vi "Found shot match.vi"(8 "error in (no error)":errorcluster, 9 "Shot data":T1, 10 "Idot match record":T2, 11 "Cap Bank Server in":refnum<class "Cap Bank Server.lvclass">) -> (0 "error out":errorcluster, 3 "Cap Bank Server out":refnum<class "Cap Bank Server.lvclass">)   [LabVIEW 2015, in "Cap Bank Server.lvclass"]
uses:
  Cap Bank Server.lvclass
  Idot match record.ctl
  User Cap Bank/Labview/Library/Shot data.ctl
  File/Controls/File formats.ctl
  <vilib>/ActorFramework/Actor/Actor.lvclass/Actor.ctl
  <vilib>/ActorFramework/Message Enqueuer/Message Enqueuer.lvclass/Message Enqueuer.ctl
  Cap Bank Server.lvclass/Cap Bank Server.ctl
  Mag Lab Measure Controller Messages/Log Status Update Msg/Log Status Update Msg.lvclass/Log Status Update Msg.ctl
  <vilib>/ActorFramework/Message Enqueuer/Init from Existing Queue.vi
  <vilib>/ActorFramework/Message Enqueuer/Enqueue.vi
  <vilib>/ActorFramework/Message Priority Queue/Priority Enqueue.vi
  <vilib>/ActorFramework/Message Enqueuer/Message Enqueuer.lvclass
  Mag Lab Measure Controller Messages/Log Status Update Msg/Log Status Update Msg.lvclass
  <vilib>/ActorFramework/Actor/Actor.lvclass
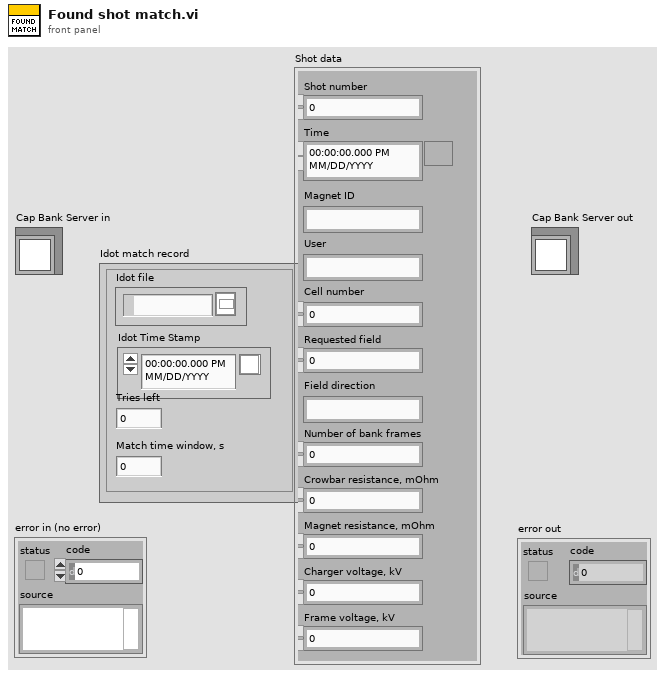
[diagram p1: front panel]
types:
  T1 = typedef "Shot data.ctl" = cluster{"Shot number":i32, "Time":timestamp, "Magnet ID":string, "User":string, "Cell number":i32, "Requested field":dbl, "Field direction":string, "Number of bank frames":i32, "Crowbar resistance, mOhm":dbl, "Magnet resistance, mOhm":dbl, "Charger voltage, kV":dbl, "Frame voltage, kV":dbl}
  T2 = typedef "Idot match record.ctl" = cluster{"Idot file":path, "Idot Time Stamp":timestamp, "Tries left":i32, "Match time window, s":dbl}
  T3 = typedef "File formats.ctl" = enum16{"TDMS", "ASCII", "BINARY"}
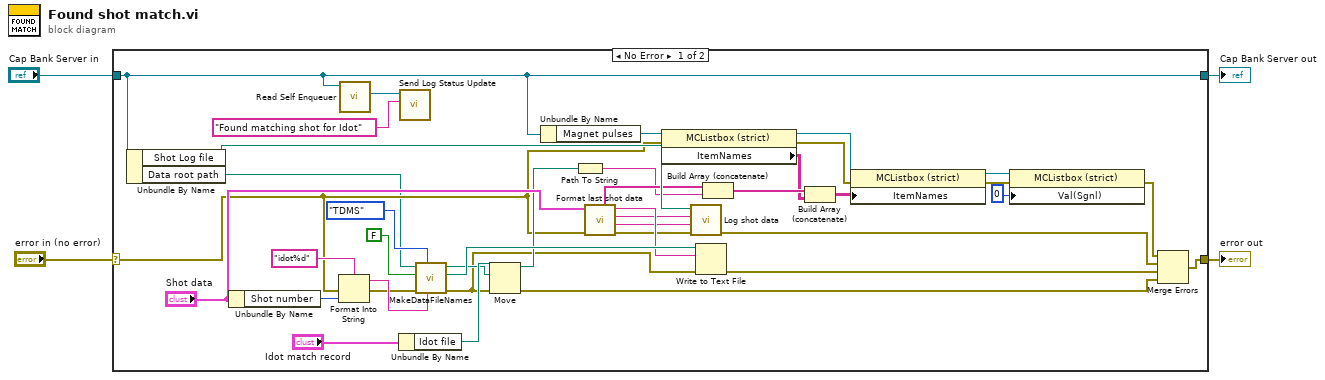
[diagram p0: block diagram]
diagram:
  n1 = case shown="No Error" "error in (no error)" {
    selector: "error in (no error)" -> [w13 w45]
    tunnel: [w26 w45] -> w3
    tunnel: [w23 w44] -> w1
    tunnel: "Cap Bank Server in" -> [w23 w44]
    frame No Error {
      n2 = Unbundle By Name(w23) -> ("Shot Log file"=w29:path, "Data root path"=w5:path)
      n3 = Unbundle By Name("Shot data") -> ("Shot number"=w34:i32)
      n4 = Format Into String(format string="idot%d", error in=w13, w34) -> (resulting string=w41:string, error out=w35:errorcluster)  [unwired: 1 in]
      n5 = call <vilib>:"Read Self Enqueuer.vi"("Actor"=w23) -> ("Self Enqueuer"=w25:refnum<class "Message Enqueuer.lvclass">)  [unwired: 10 in]
      n6 = Unbundle By Name("Idot match record") -> ("Idot file"=w32:path)
      n7 = call "Send Log Status Update.vi"("Status"="Found matching shot for Idot", "Message Enqueuer"=w25) -> ()  [unwired: 8 in, 2 out]
      n8 = call "MakeDataFileNames.vi"("File Prefix"=w41, "File format"=File_formats."TDMS", "Error In"=w35, "Generate Index"=FALSE, "Root Data Folder"=w5) -> ("Error Out"=w16:errorcluster, "Settings File Path"=w39:path, "Data File  Path"=w31:path)  [unwired: 3 in, 1 out]
      n9 = Move(source path=w32, error in=w16, 10:w31) -> (error out=w27:errorcluster, 3:w21:path)  [unwired: 2 in, 1 out]
      n10 = Unbundle By Name(w23) -> ("Magnet pulses"=w22:refnum<vi>)
      n11 = Path To String(path=w21) -> (string=w19:string)
      n12 = call "Format last shot data.vi"("error in (no error)"=w13, "Shot data"="Shot data") -> ("error out"=w15:errorcluster, "Spreadsheet header string"=w36:string, "Spreadsheet shot string"=w37:string, "Formated shot data"=w38:string, "Listbox entry"=w20:string[])  [unwired: 5 in]
      n13 = property class="MCListbox (strict)"(reference=w22, error in=w13) -> (reference out=w18:refnum<vi>, error out=w17:errorcluster, "ItemNames"=w11:string[][])
      n14 = call "Log shot data.vi"("error in (no error)"=w15, "Spreadsheet header string"=w36, "Spreadsheet shot string"=w37, "Log file folder"=w29) -> ("error out"=w14:errorcluster)  [unwired: 6 in, 1 out]
      n15 = Write to Text File(file (use dialog)=w39, text=w38, error in=w16) -> (error out=w28:errorcluster)  [unwired: 1 in, 2 out]
      n16 = Build Array (concatenate)(w20, w19) -> (w12:string[])
      n17 = Build Array (concatenate)(w12, w11) -> (w10:string[][])
      n18 = property class="MCListbox (strict)"(reference=w18, error in=w17, "ItemNames"=w10) -> (reference out=w9:refnum<vi>, error out=w7:errorcluster)
      n19 = property class="MCListbox (strict)"(reference=w9, error in=w7, "Val(Sgnl)"=0 ("Value (Signaling)")) -> (error out=w6:errorcluster)  [unwired: 1 out]
      n20 = Merge Errors(w6, w14, w28, w27) -> (w26:errorcluster)
    }
    frame Error {
    }
  }
  "error out" <- w3
  "Cap Bank Server out" <- w1
